vi "AttackerBlockSkill.vi"(6 "Attack ourselves":bool, 8 "error in (no error)":errorcluster, 9 "Game":refnum<class "Game.lvclass">, 10 "Robot":refnum<class "Robot.lvclass">, 11 "AttackerBlockSkill in":refnum<class "AttackerBlockSkill.lvclass">) -> (0 "error out":errorcluster, 2 "Robot out":refnum<class "Robot.lvclass">, 3 "AttackerBlockSkill out":refnum<class "AttackerBlockSkill.lvclass">)   [LabVIEW 2018, in "AttackerBlockSkill.lvclass"]
uses:
  AttackerBlockSkill.lvclass
  Robot_class/Robot.lvclass
  Game_class/Game.lvclass
  Game_class/Game.lvclass/Game.ctl
  Object_class/Object.lvclass/Object.ctl
  Robot_class/Robot.lvclass/Robot.ctl
  <vilib>/Analysis/_algsub.llb/Real Vector Norm.vi
  Game_class/Read BallRef.vi
  Game_class/Read FieldRef.vi
  Object_class/Read x.vi
  Object_class/Read y.vi
  Robot_class/Write dest_x.vi
  Robot_class/Write dest_y.vi
  Robot_class/Write dest_orientation.vi
  Ball_class/Ball.lvclass
  C:/Users/Rebeca/Documents/Rebeca/Roboime/SSL_AI - Carla/Object_class/Object.lvclass
  Field_class/Field.lvclass
  <vilib>/Analysis/NI_AALPro.lvlib
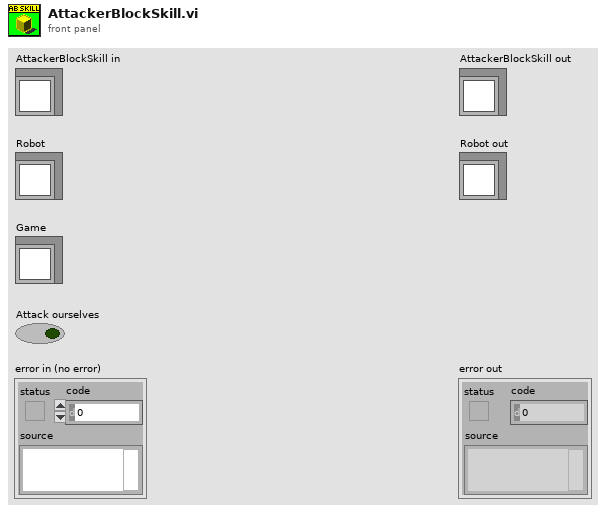
[diagram p1: front panel]
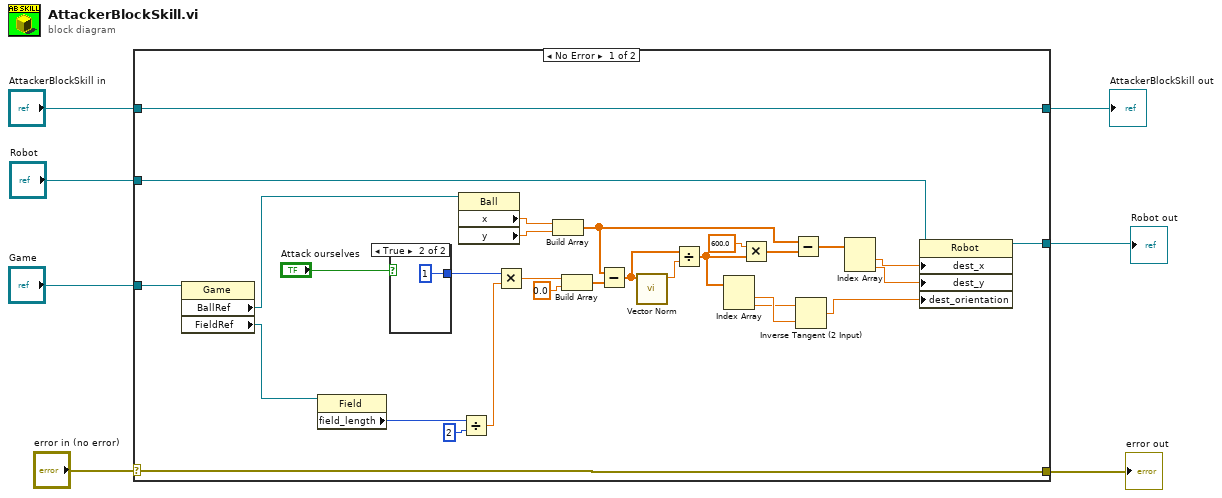
[diagram p0: block diagram]
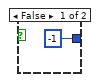
[diagram p2: hidden frame]
diagram:
  n1 = case shown="No Error" "error in (no error)" {
    selector: "error in (no error)" -> [w35 w41]
    tunnel: [w35 w41] -> w6
    tunnel: [w36 w40] -> w4
    tunnel: "AttackerBlockSkill in" -> [w36 w40]
    tunnel: "Robot" -> [w19 w39]
    tunnel: "Game" -> [w18 _]
    tunnel: [w34 w39] -> w1
    frame No Error {
      n2 = property class="Game"(reference=w18) -> ("BallRef"=w15:refnum<class "Ball.lvclass">, "FieldRef"=w17:refnum<class "Field.lvclass">)  [unwired: 1 in, 2 out]
      n3 = property class="Field"(reference=w17) -> ("field_length"=w16:i32)  [unwired: 1 in, 2 out]
      n4 = case shown="True" "Attack ourselves" {
        tunnel: [-1 1] -> w30
        frame False {
        }
        frame True {
        }
      }
      n5 = property class="Ball"(reference=w15) -> ("x"=w14:dbl, "y"=w13:dbl)  [unwired: 1 in, 2 out]
      n6 = Divide(x=w16, y=u32 2) -> (x/y=w32:dbl)
      n7 = Multiply(x=w30, y=w32) -> (x*y=w29:dbl)
      n8 = Build Array(w14, w13) -> (w31:dbl[])
      n9 = Build Array(w29, 0.0 ("element")) -> (w25:dbl[])
      n10 = Subtract(x=w31, y=w25) -> (x-y=w26:dbl[])
      n11 = call-poly <vilib>:"Vector Norm.vi"("Input Vector"=w26) -> ("norm"=w27:dbl)  [unwired: 9 in, 1 out]
      n12 = Divide(x=w26, y=w27) -> (x/y=w22:dbl[])
      n13 = Index Array(array=w22) -> (element #1=w24:dbl, element #2=w23:dbl)  [unwired: 2 in]
      n14 = Multiply(x=600.0, y=w22) -> (x*y=w20:dbl[])
      n15 = Subtract(x=w31, y=w20) -> (x-y=w12:dbl[])
      n16 = Inverse Tangent (2 Input)(1:w24, 2:w23) -> (0:w9:dbl)
      n17 = Index Array(array=w12) -> (element #1=w11:dbl, element #2=w10:dbl)  [unwired: 2 in]
      n18 = property class="Robot"(reference=w19, "dest_x"=w11, "dest_y"=w10, "dest_orientation"=w9) -> (reference out=w34:refnum<class "Robot.lvclass">)  [unwired: 1 in, 1 out]
    }
    frame Error {
    }
  }
  "error out" <- w6
  "AttackerBlockSkill out" <- w4
  "Robot out" <- w1
